vi "readWithPreamble.vi"() -> ()   [LabVIEW 2013]
uses:
  <vilib>/Instr/_visa.llb/VISA Configure Serial Port (Instr).vi
panel:
  out "input byte data":u8[][](array[numeric])
  out "counter":i32[](array[numeric])
  out "state":i32[](array[numeric])
  in  "stop":bool
  in  "state":i32
  in  "dataCounter":i32
  out "cell":u8[](array[numeric])
  out "output_int16":i32[](array[numeric])
  in  "baud rate":u32=9600
  in  "serial_port":refnum<visa-resource-name> caption="Porta Serial"
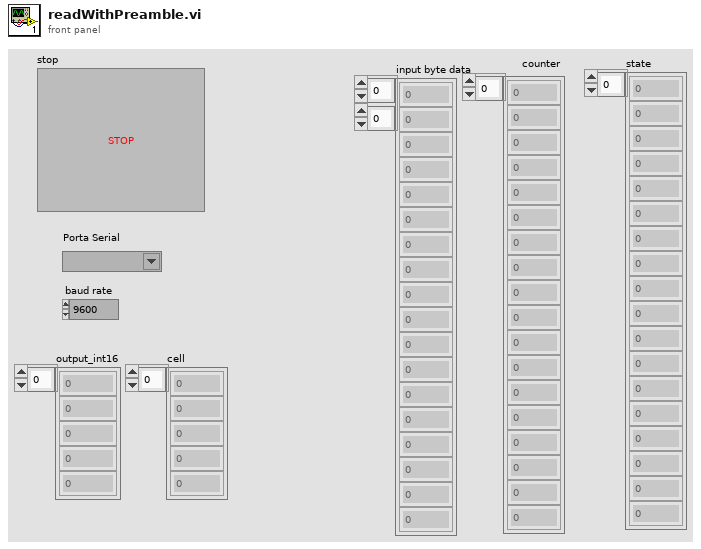
[diagram p1: front panel]
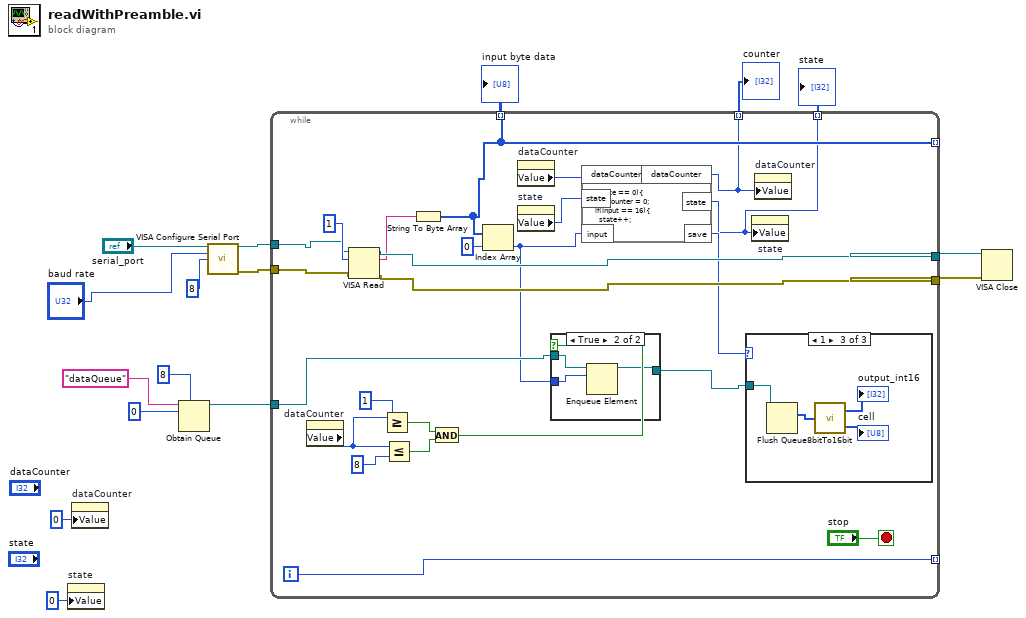
[diagram p0: block diagram]
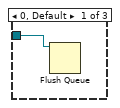
[diagram p2: hidden frame]
diagram:
  n1 = property on="state" class="DigNum (strict)"("Value"=0 ("state")) -> ()  [unwired: 2 in, 2 out]
  n2 = property on="dataCounter" class="DigNum (strict)"("Value"=0 ("dataCounter")) -> ()  [unwired: 2 in, 2 out]
  n3 = Obtain Queue(max queue size (-1, unlimited)=8, name (unnamed)="dataQueue", element data type=u8 0) -> (queue out=w3:refnum<queue>)  [unwired: 2 in, 2 out]
  n4 = call-poly "VISA Configure Serial Port"("VISA resource name"="serial_port", "baud rate (9600)"="baud rate", "data bits (8)"=u16 8) -> ("VISA resource name out"=w14:refnum<visa-resource-name>, "error out"=w13:errorcluster)  [unwired: 11 in]
  n5 = while {
    tunnel: w14 -> [w38]
    tunnel: w13 -> [w39]
    tunnel: [w36] -> w12
    tunnel: [w37] -> w11
    tunnel: [w34] -> _ mode=indexing
    tunnel: [w27] -> _ mode=indexing
    tunnel: [w27] -> w7 mode=indexing
    tunnel: w3 -> [w24]
    tunnel: [w18] -> w2 mode=indexing
    tunnel: [w17] -> w1 mode=indexing
    i -> [w34]
    stop <- "stop" stop-if-true
    n6 = property on="dataCounter" class="DigNum (strict)"() -> ("Value"=w26:i32)  [unwired: 2 in, 2 out]
    n7 = VISA Read(VISA resource name=w38, byte count=1, error in (no error)=w39) -> (VISA resource name out=w37:refnum<visa-resource-name>, read buffer=w35:string, error out=w36:errorcluster)  [unwired: 1 out]
    n8 = Greater Or Equal?(x=w26, y=1) -> (x >= y?=w33:bool)
    n9 = Less Or Equal?(x=w26, y=8) -> (x <= y?=w32:bool)
    n10 = String To Byte Array(string=w35) -> (unsigned byte array=w27:u8[])
    n11 = And(x=w33, y=w32) -> (x .and. y?=w31:bool)
    n12 = Index Array(array=w27, index=0) -> (element=w21:u8)
    n13 = property on="dataCounter" class="DigNum (strict)"() -> ("Value"=w23:i32)  [unwired: 2 in, 2 out]
    n14 = property on="state" class="DigNum (strict)"() -> ("Value"=w22:i32)  [unwired: 2 in, 2 out]
    n15 = case shown="True" w31 {
      tunnel: w21 -> [_ w48]
      tunnel: w24 -> [w46 w49]
      tunnel: [w46 w47] -> w19
      frame False {
      }
      frame True {
        n16 = Enqueue Element(queue=w49, element=w48) -> (queue out=w47:refnum<queue>)  [unwired: 2 in, 2 out]
      }
    }
    n17 = formula code="int save = 2;\n\nif(state == 0){\ndataCounter = 0;\n  if(input == 16){\n    state++;\n  }\n}\nelse if(state == 1){\n  if(input == 32){\n      state ++;\n}\n  else{\n      state = 0;\n}\n}\nelse if(state == 2){\n  if(input == 64 ){\n     state++;\n}\n   else{\n     dataCounter++;\n}\n}\nelse if (state == 3){\n  if(input == 128 && dataCounter == 7){\n    save = 1;\n  }else\n{\n    save = 0;\n}\n state = 0;\n}"("input"=w21, "state"=w22, "dataCounter"=w23) -> ("dataCounter"=w18:i32, "state"=w17:i32, "save"=w20:i32)
    n18 = case shown="1" w20 {
      tunnel: w19 -> [w41 _ w43]
      frame 0, Default {
        n19 = Flush Queue(queue=w41) -> ()  [unwired: 1 in, 3 out]
      }
      frame 2 {
      }
      frame 1 {
        n20 = Flush Queue(queue=w43) -> (remaining elements=w42:u8[])  [unwired: 1 in, 2 out]
        n21 = call "8bitTo16bit.vi"("input_byte"=w42) -> ("output_int16"=→"output_int16":i32[], "cell"=→"cell":u8[])
      }
    }
    n22 = property on="state" class="DigNum (strict)"("Value"=w17) -> ()  [unwired: 2 in, 2 out]
    n23 = property on="dataCounter" class="DigNum (strict)"("Value"=w18) -> ()  [unwired: 2 in, 2 out]
  }
  "state" <- w1
  "counter" <- w2
  "input byte data" <- w7
  n24 = VISA Close(VISA resource name=w11, error in (no error)=w12) -> ()  [unwired: 1 out]
